vi "散斑图像作用.vi"(10 "图像簇":T1, 11 "光源散斑簇":T2) -> (3 "散斑图像作用聚焦数组":dbl[](array[numeric]))   [LabVIEW 2018]
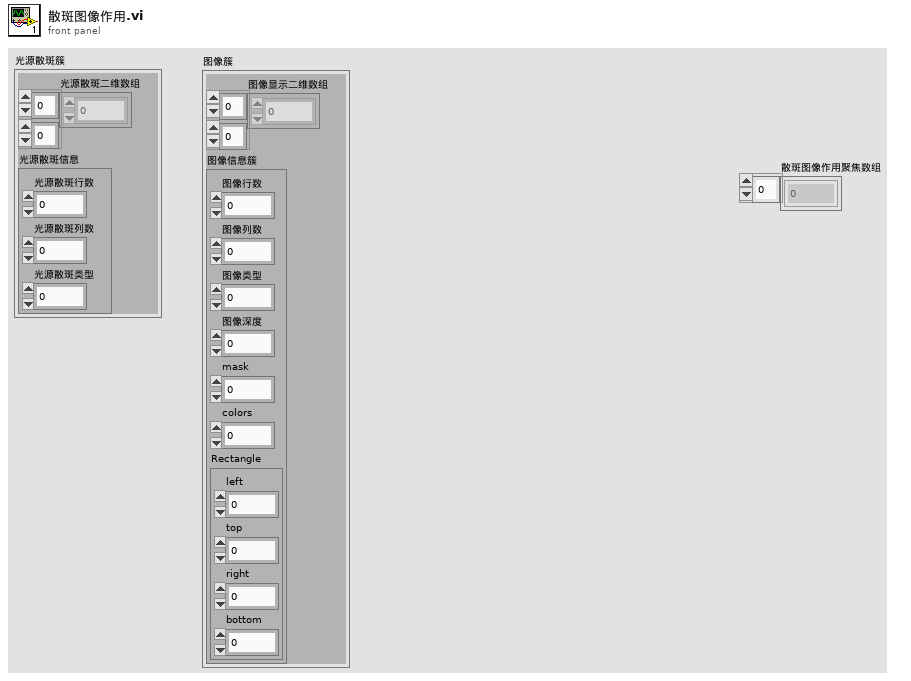
[diagram p1: front panel]
types:
  T1 = cluster{"图像显示二维数组":dbl[][], "图像信息簇":cluster{"图像行数":dbl, "图像列数":dbl, "图像类型":dbl, "图像深度":i32, "mask":i32, "colors":i32, "Rectangle":cluster{"left":i16, "top":i16, "right":i16, "bottom":i16}}}
  T2 = cluster{"光源散斑二维数组":dbl[][], "光源散斑信息":cluster{"光源散斑行数":dbl, "光源散斑列数":dbl, "光源散斑类型":dbl}}
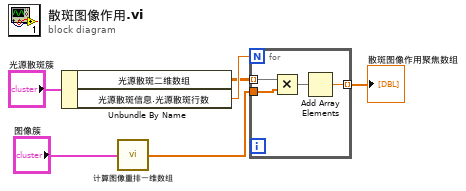
[diagram p0: block diagram]
diagram:
  n1 = Unbundle By Name("光源散斑簇") -> ("光源散斑二维数组"=w3:dbl[][], "光源散斑信息.光源散斑行数"=w4:dbl)
  n2 = call "计算图像重排一维数组.vi"("优化图像簇"="图像簇") -> ("图像重排一维数组"=w1:dbl[])
  n3 = for {
    N: w4 -> [_]
    tunnel: w3 -> [w10] mode=indexing
    tunnel: w1 -> [w9]
    tunnel: [w7] -> w6 mode=indexing
    n4 = Multiply(x=w10, y=w9) -> (x*y=w8:dbl[])
    n5 = Add Array Elements(numeric array=w8) -> (sum=w7:dbl)
  }
  "散斑图像作用聚焦数组" <- w6
